vi "TS DotStar SPI V5 - Switched Style.vi"() -> ()   [LabVIEW 2016]
doc: "ADXL362 SPI Accelerometer\n\nThis example shows how to use the Analog Devices ADXL362 Accelerometer sensor connected to SPI.\n\nThis example expects a USB cable connected from your development PC to the Type B USB Jack (next to the power input) on the roboRIO."
uses:
  <vilib>/Rock Robotics/SystemInterfaces/spilib/spi_bus.ctl
  <vilib>/Rock Robotics/WPI/SPI/WPI_SPIMode.ctl
panel:
  out "ONOFF":bool
  in  "Blink Rate":u32
  in  "Aiming":u32(colorbox)
  in  "Loader":bool
  in  "Intake":bool
  in  "Shooter":bool
  in  "Blinky End":u8
  in  "Chaser (Gap)":u8
  in  "Display Style":u8(knob) scale=0.0..6.0
  out "Aiming":bool
  out "Loader":bool
  out "Intake":bool
  out "Shooter":bool
  in  "Global Max\nBrightness":u8(slide) max=31 scale=0.0..31.0
  in  "Brightness B":u8
  in  "Brighness R":u8
  in  "Brigtness G":u8
  in  "Blue":bool
  in  "Red":bool
  in  "Green":bool
  in  "Number of Lights":u8
  in  "Number ON":u8
  in  "Chip Select Active High (F)":bool
  in  "Mode (3)":T1=enum."Mode 3 (Clk Idle High,Sample on Trailing)"
  in  "Clock Rate (Hz)":dbl=500000.0
  in  "error in":errorcluster
  in  "SPI Bus":T2=enum."SPI On-Board, CS1"
  out "error out":errorcluster
  in  "stop":bool
  # "Set these inputs before running."
  # "Number of Lights"
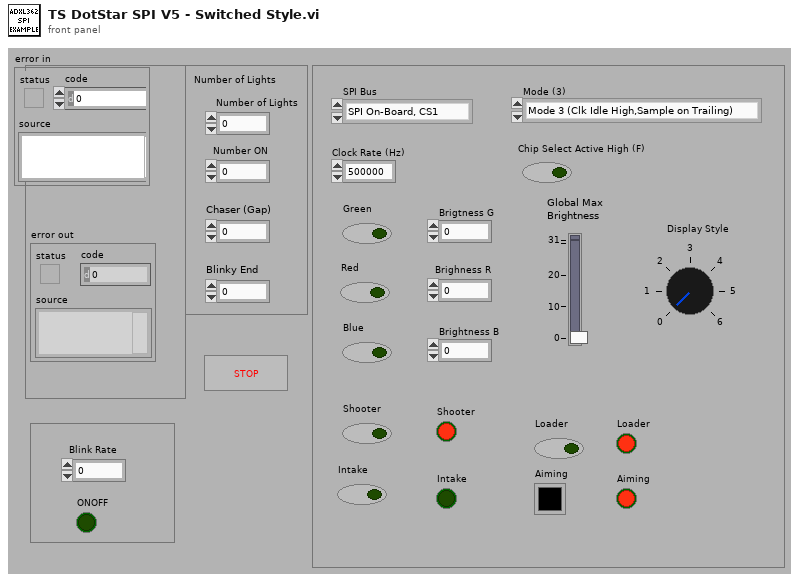
[diagram p1: front panel]
types:
  T1 = typedef "WPI_SPIMode.ctl" = enum16{"Mode 0 (Clk Idle Low,Sample on Leading)", "Mode 1 (Clk Idle Low,Sample on Trailing)", "Mode 2 (Clk Idle High,Sample on Leading)", "Mode 3 (Clk Idle High,Sample on Trailing)"}
  T2 = typedef "spi_bus.ctl" = enum16{"SPI On-Board, CS0", "SPI On-Board, CS1", "SPI On-Board, CS2", "SPI On-Board, CS3", "SPI MXP", "Invalid"}
  T3 = typedef "WPI_SPIDevRef.ctl" = cluster{"DevStatus":errorcluster, "Handle":i32, "SPI Bus":T2}
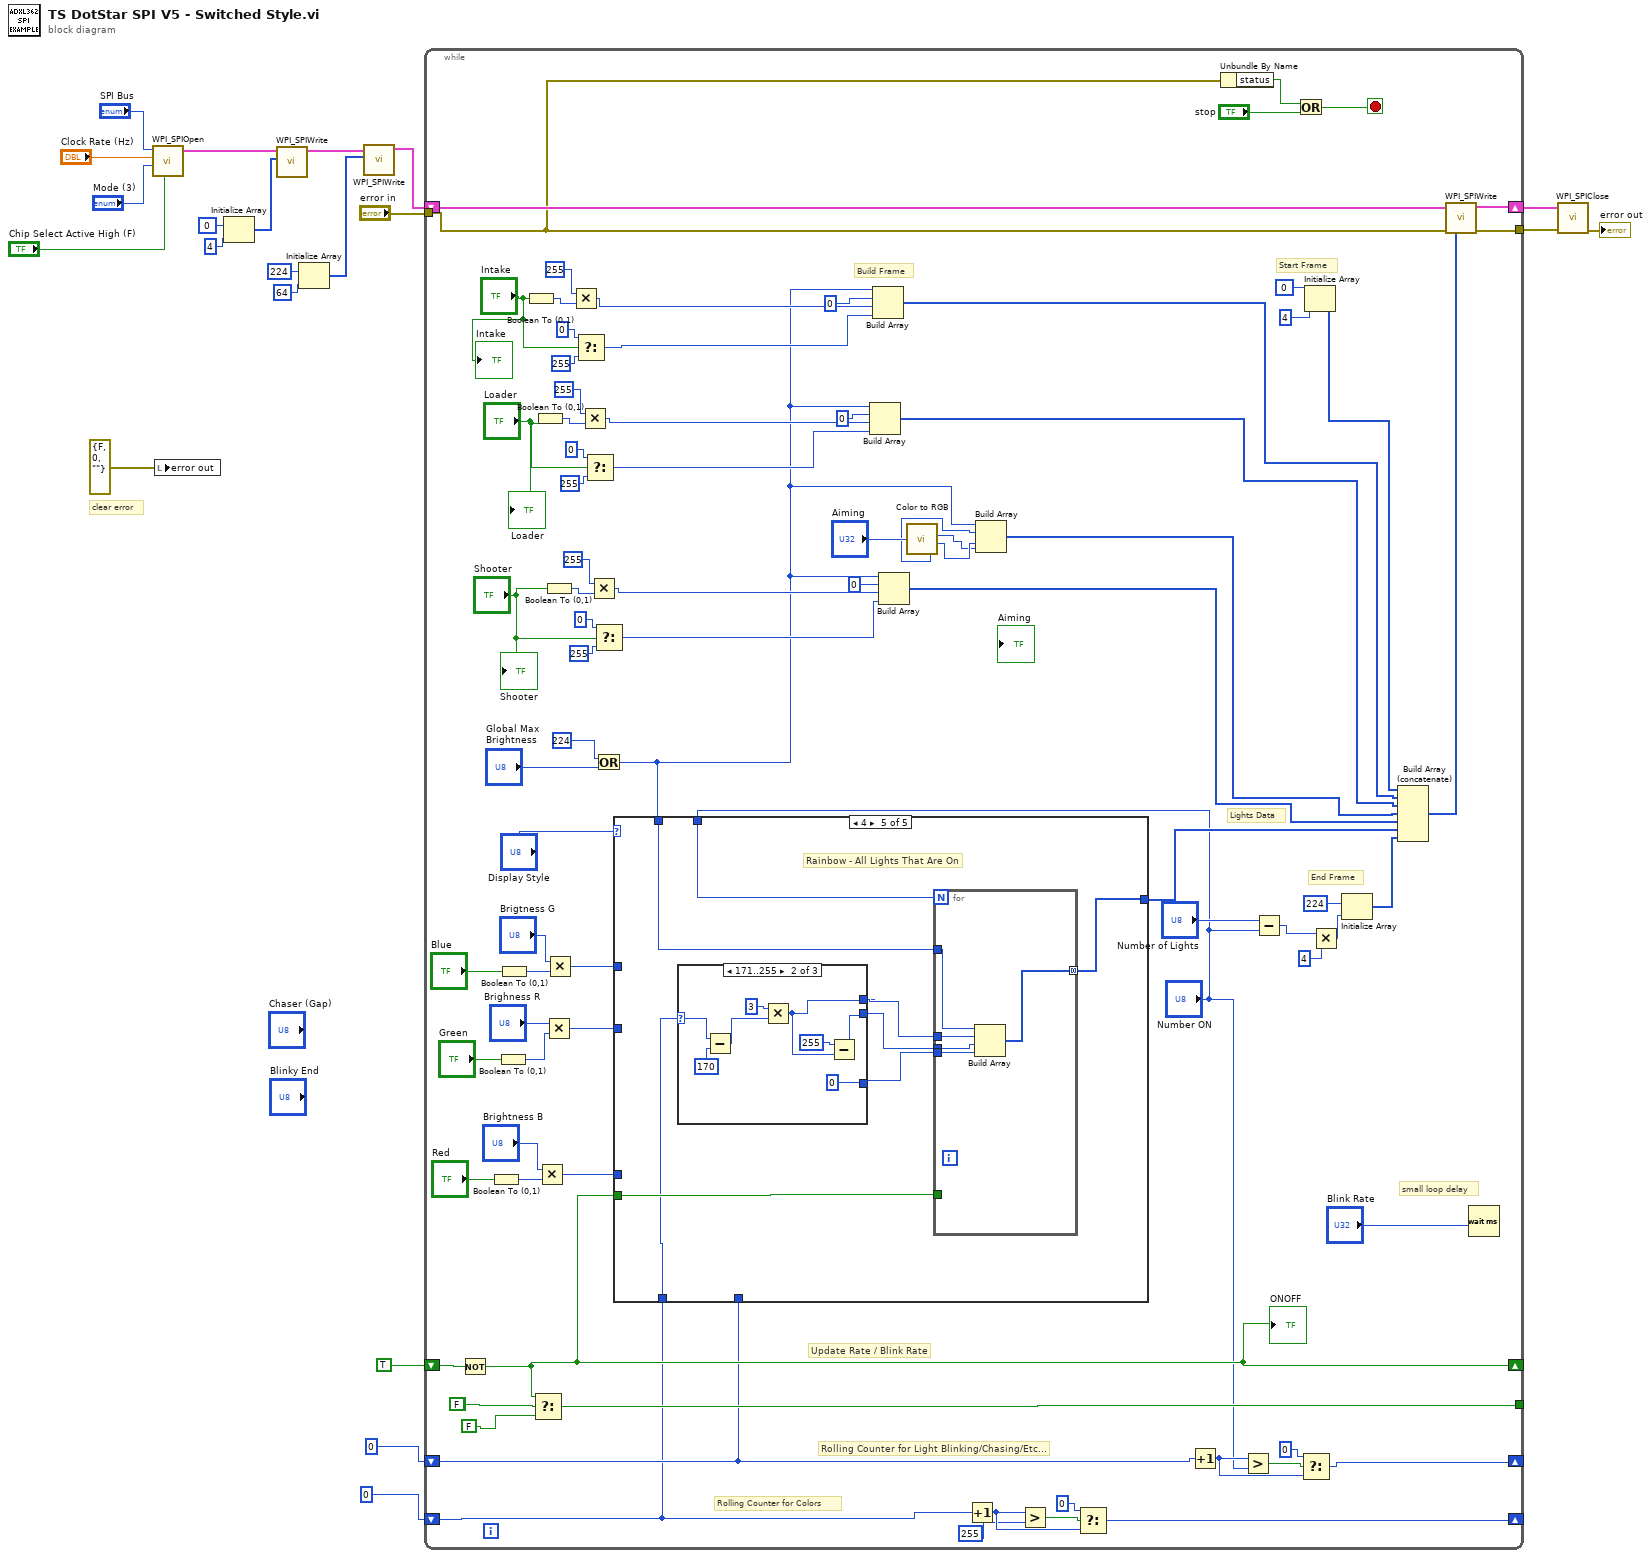
[diagram p0: block diagram]
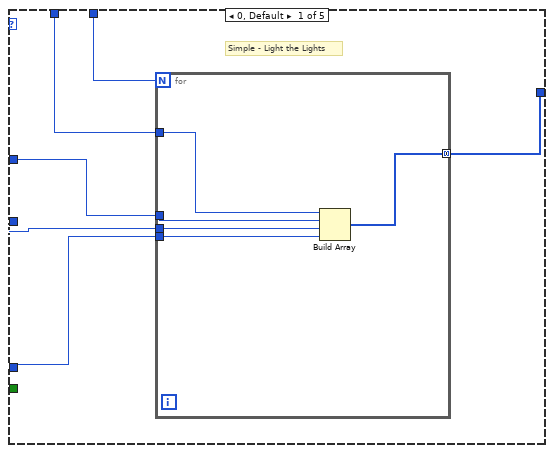
[diagram p2: hidden frame]
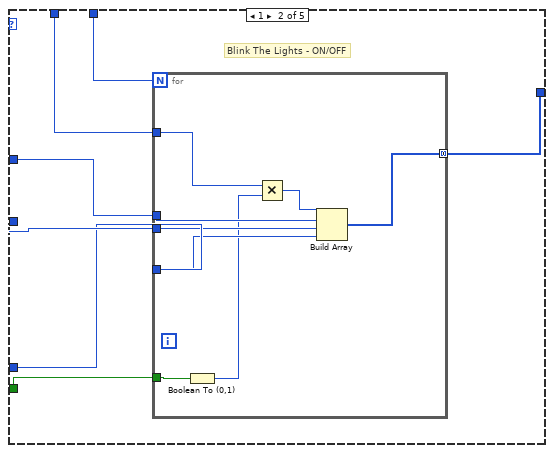
[diagram p3: hidden frame]
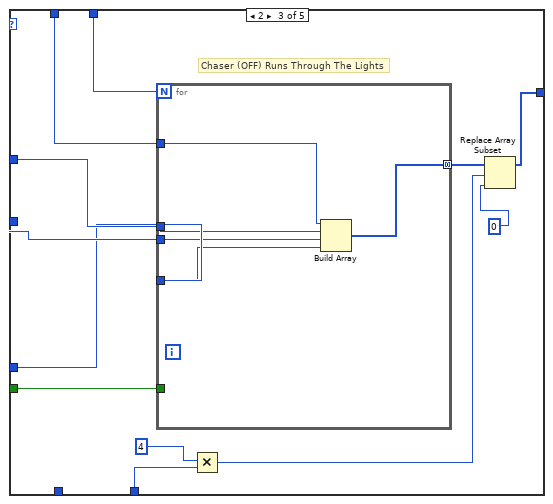
[diagram p4: hidden frame]
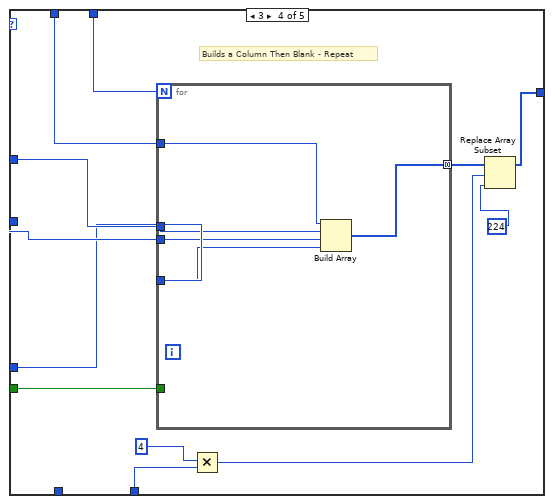
[diagram p5: hidden frame]
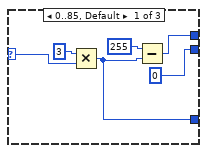
[diagram p6: hidden frame]
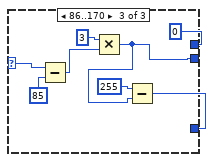
[diagram p7: hidden frame]
diagram:
  # "clear error"
  n1 = call <vilib>:"WPI_SPIOpen.vi"("Chip Select Active High (F)"="Chip Select Active High (F)", "Mode (3)"="Mode (3)", "Clock Rate (Hz)"="Clock Rate (Hz)", "SPI Bus"="SPI Bus") -> ("SPIDevRef"=w11:T3)  [unwired: 6 in, 1 out]
  n2 = local write "error out"(errorcluster {"status"=FALSE, "code"=0, "source"=""} ("error out")) -> ()
  n3 = Initialize Array(u8 0 ("Data To Send"), u8 4 ("dimension size")) -> (w10:u8[])
  n4 = call <vilib>:"WPI_SPIWrite.vi"("Data To Send"=w10, "SPIDevRef"=w11) -> ("SPIDevRef"=w4:T3)  [unwired: 7 in, 2 out]
  n5 = Initialize Array(u8 224 ("Data To Send"), u8 64 ("dimension size")) -> (w6:u8[])
  n6 = call <vilib>:"WPI_SPIWrite.vi"("Data To Send"=w6, "SPIDevRef"=w4) -> ("SPIDevRef"=w9:T3)  [unwired: 7 in, 2 out]
  n7 = while {
    shift-right: [w101] -> w18
    shift-left: w9 -> [w93]
    tunnel: "error in" -> [w89]
    tunnel: [w100] -> w5
    tunnel: [w36] -> _
    shift-right: [w34] -> _
    shift-left: TRUE -> [w35]
    shift-right: [w30] -> _
    shift-left: 0 -> [w28]
    shift-right: [w24] -> _
    shift-left: 0 -> [w22]
    stop <- w88 stop-if-true
    (unwired) TRUE
    # "Update Rate / Blink Rate"
    # "Rolling Counter for Light Blinking/Chasing/Etc..."
    # "Rolling Counter for Colors"
    # "Build Frame"
    # "Lights Data"
    # "End Frame"
    # "Start Frame"
    # "small loop delay"
    n8 = Not(x=w35) -> (.not. x?=w34:bool)
    "ONOFF" <- w34
    n9 = Boolean To (0,1)(Boolean="Red") -> (0, 1=w46:i16)
    n10 = Boolean To (0,1)(Boolean="Green") -> (0, 1=w47:i16)
    n11 = Boolean To (0,1)(Boolean="Blue") -> (0, 1=w48:i16)
    n12 = Boolean To (0,1)(Boolean="Intake") -> (0, 1=w85:i16)
    n13 = Select(t=w34, s=FALSE, f=FALSE) -> (s? t:f=w36:bool)
    n14 = Boolean To (0,1)(Boolean="Loader") -> (0, 1=w78:i16)
    n15 = Multiply(x="Brightness B", y=w46) -> (x*y=w41:i16)
    n16 = Boolean To (0,1)(Boolean="Shooter") -> (0, 1=w73:i16)
    n17 = Multiply(x="Brighness R", y=w47) -> (x*y=w42:i16)
    n18 = Multiply(x="Brigtness G", y=w48) -> (x*y=w40:i16)
    n19 = Multiply(x=u8 255, y=w85) -> (x*y=w67:i16)
    n20 = Select(t=u8 0, s="Intake", f=u8 255) -> (s? t:f=w68:u8)
    n21 = Multiply(x=u8 255, y=w78) -> (x*y=w65:i16)
    n22 = Select(t=u8 0, s="Loader", f=u8 255) -> (s? t:f=w64:u8)
    n23 = Multiply(x=u8 255, y=w73) -> (x*y=w62:i16)
    n24 = Select(t=u8 0, s="Shooter", f=u8 255) -> (s? t:f=w61:u8)
    n25 = Or(x=u8 224, y="Global Max\nBrightness") -> (x .or. y?=w52:u8)
    n26 = case shown="4" "Display Style" {
      tunnel: [w111 w123 w134 w151 w170] -> w53
      tunnel: w52 -> [w110 w122 w143 w160 w173]
      tunnel: "Number ON" -> [w109 w121 w138 w155 w171]
      tunnel: w42 -> [w107 w119 w141 w158 _]
      tunnel: w41 -> [w106 w118 w140 w157 _]
      tunnel: w40 -> [w108 w120 w142 w159 _]
      tunnel: w34 -> [_ w117 w139 w156 w172]
      tunnel: w28 -> [_ _ w137 w154 _]
      tunnel: w22 -> [_ _ _ _ w169]
      frame 0, Default {
        # "Simple - Light the Lights"
        n27 = for {
          N: w109 -> [_]
          tunnel: [w116] -> w111 mode=concatenating
          tunnel: w110 -> [w115]
          tunnel: w108 -> [w114]
          tunnel: w107 -> [w113]
          tunnel: w106 -> [w112]
          n28 = Build Array(w115, w114, w113, w112) -> (w116:i16[])
        }
      }
      frame 1 {
        # "Blink The Lights - ON/OFF"
        n29 = for {
          N: w121 -> [_]
          tunnel: [w131] -> w123 mode=concatenating
          tunnel: w122 -> [w126]
          tunnel: w120 -> [w130]
          tunnel: w119 -> [w129]
          tunnel: w118 -> [w128]
          tunnel: w117 -> [w127]
          n30 = Boolean To (0,1)(Boolean=w127) -> (0, 1=w125:i16)
          n31 = Multiply(x=w126, y=w125) -> (x*y=w124:i16)
          n32 = Build Array(w124, w130, w129, w128) -> (w131:i16[])
        }
      }
      frame 2 {
        # "Chaser (OFF) Runs Through The Lights"
        n33 = for {
          N: w138 -> [_]
          tunnel: [w148] -> w135 mode=concatenating
          tunnel: w143 -> [w144]
          tunnel: w142 -> [w147]
          tunnel: w141 -> [w146]
          tunnel: w140 -> [w145]
          tunnel: w139 -> [_]
          n34 = Build Array(w144, w147, w146, w145) -> (w148:i16[])
        }
        n35 = Multiply(x=4, y=w137) -> (x*y=w133:i32)
        n36 = Replace Array Subset(array=w135, new element=u8 0, index=w133) -> (w134:i16[])
      }
      frame 3 {
        # "Builds a Column Then Blank - Repeat"
        n37 = for {
          N: w155 -> [_]
          tunnel: [w165] -> w152 mode=concatenating
          tunnel: w160 -> [w161]
          tunnel: w159 -> [w164]
          tunnel: w158 -> [w163]
          tunnel: w157 -> [w162]
          tunnel: w156 -> [_]
          n38 = Build Array(w161, w164, w163, w162) -> (w165:i16[])
        }
        n39 = Multiply(x=4, y=w154) -> (x*y=w150:i32)
        n40 = Replace Array Subset(array=w152, new element=u8 224, index=w150) -> (w151:i16[])
      }
      frame 4 {
        # "Rainbow - All Lights That Are On"
        n41 = case shown="171..255" w169 {
          selector: w169 -> [w175 w184 w193]
          tunnel: [w177 w180 0] -> w168
          tunnel: [0 w182 w188] -> w167
          tunnel: [w174 0 w189] -> w166
          frame 0..85, Default {
            n42 = Multiply(x=3, y=w175) -> (x*y=w174:i32)
            n43 = Subtract(x=255, y=w174) -> (x-y=w177:i32)
          }
          frame 171..255 {
            n44 = Subtract(x=w184, y=170) -> (x-y=w181:i32)
            n45 = Multiply(x=3, y=w181) -> (x*y=w180:i32)
            n46 = Subtract(x=255, y=w180) -> (x-y=w182:i32)
          }
          frame 86..170 {
            n47 = Subtract(x=w193, y=85) -> (x-y=w190:i32)
            n48 = Multiply(x=3, y=w190) -> (x*y=w188:i32)
            n49 = Subtract(x=255, y=w188) -> (x-y=w189:i32)
          }
        }
        n50 = for {
          N: w171 -> [_]
          tunnel: [w200] -> w170 mode=concatenating
          tunnel: w173 -> [w199]
          tunnel: w172 -> [_]
          tunnel: w168 -> [w198]
          tunnel: w167 -> [w197]
          tunnel: w166 -> [w196]
          n51 = Build Array(w199, w198, w197, w196) -> (w200:i32[])
        }
      }
    }
    n52 = Build Array(w52, u8 0, w65, w64) -> (w75:i16[])
    n53 = Build Array(w52, u8 0, w67, w68) -> (w81:i16[])
    n54 = Build Array(w52, u8 0, w62, w61) -> (w70:i16[])
    n55 = call <vilib>:"Color to RGB.vi"("Color"="Aiming") -> ("R"=w58:u8, "G"=w59:u8, "B"=w60:u8)  [unwired: 1 out]
    n56 = Increment(x=w22) -> (x+1=w25:u8)
    n57 = Build Array(w52, w60, w59, w58) -> (w80:u8[])
    n58 = Greater?(x=w25, y=255) -> (0:w26:bool)
    n59 = Select(t=0, s=w26, f=w25) -> (s? t:f=w24:i32)
    n60 = Increment(x=w28) -> (x+1=w31:u8)
    n61 = Unbundle By Name(w89) -> ("status"=w90:bool)
    n62 = Greater?(x=w31, y="Number ON") -> (0:w32:bool)
    n63 = Subtract(x="Number of Lights", y="Number ON") -> (x-y=w94:u8)
    n64 = Or(x=w90, y="stop") -> (x .or. y?=w88:bool)
    n65 = Select(t=0, s=w32, f=w31) -> (s? t:f=w30:i32)
    n66 = Initialize Array(u8 0 ("Data To Send"), u8 4 ("dimension size")) -> (w82:u8[])
    n67 = Multiply(x=w94, y=u8 4 ("dimension size")) -> (x*y=w96:u8)
    n68 = Initialize Array(u8 224 ("Data To Send"), w96) -> (w92:u8[])
    n69 = Build Array (concatenate)(w82, w81, w75, w80, w70, w53, w92) -> (w91:i32[])
    n70 = call <vilib>:"WPI_SPIWrite.vi"("error in (no error)"=w89, "Data To Send"=w91, "SPIDevRef"=w93) -> ("error out"=w100:errorcluster, "SPIDevRef"=w101:T3)  [unwired: 6 in, 1 out]
    n71 = Wait (ms)(milliseconds to wait="Blink Rate") -> ()  [unwired: 1 out]
    "Shooter" <- "Shooter"
    "Loader" <- "Loader"
    "Intake" <- "Intake"
  }
  n72 = call <vilib>:"WPI_SPIClose.vi"("error in (no error)"=w5, "SPIDevRef"=w18) -> ("error out"=→"error out":errorcluster)  [unwired: 9 in]
